vi "Open Front Panel.vi"(8 "error in":errorcluster, 11 "Session In":T1) -> (0 "error out":errorcluster, 3 "Session Out":T1)   [LabVIEW 2015, in "System Log.lvclass"]
uses:
  System Log.lvclass
  <userlib>/_Session Fwk/Typedefs/Session Handle.ctl
  <userlib>/_Session Fwk/Session - Root.lvclass
  Controls/DVR.ctl
  System Log.lvclass/System Log.ctl
  Accessors/Read Log VI.vi
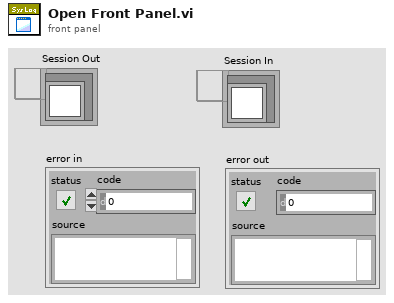
[diagram p1: front panel]
types:
  T1 = typedef "Session - Root.lvclass/Session Handle.ctl" = refnum<data-value>
  T2 = typedef "System Log.lvclass/DVR.ctl" = refnum<data-value>
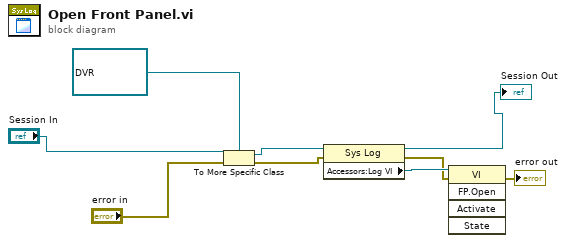
[diagram p0: block diagram]
diagram:
  n1 = To More Specific Class(target class=T2 refnum ("DVR"), reference="Session In", error in="error in") -> (specific class reference=w6:T2, error out=w4:errorcluster)
  n2 = property class="Sys Log"(reference=w6, error in=w4) -> (reference out=→"Session Out":T2, error out=w3:errorcluster, "Accessors:Log VI"=w5:refnum<vi>)
  n3 = invoke class="VI" method="FP.Open"(reference=w5, error in=w3) -> (error out=→"error out":errorcluster)  [unwired: 3 in, 4 out]
